vi "Valuta procedure start stop.vi"(6 "UTILIZZO BANCO":T1(ring), 7 "Modalità avvio":T9={"MODALITA' BANCO"=enum."ALIMENTATORE E FRENO", "MODALITA' AVVIO MOTORE"=enum."AVVIO A TENSIONE RIDOTTA", "MODALITA' AVVIO FRENO"=enum."MARCIA PRIMA AVVIO", "V avvio[V]"=0.0, "F avvio[Hz]"=0.0, "%V ridotta"=0.0, "C avvio [Nm]"=0.0, "RPM avvio"=0.0, "SERVO AVVIO"=FALSE, "SENSO DI ROTAZIONE"=FALSE}, 8 "Stato alimentatore 1":T6 {"Alimentatore 1"."Status ref"."RIF 2" scale=0.0..100.0; "Alimentatore 1"."Status ref"."RIF 1" scale=0.0..100.0}, 9 "Stato inverter":T7, 10 "NUOVO STEP":T3={"Tipo prova"="", "Misura resistenza ?"=FALSE, "Tempo Step[s]"=1.0, "Freno"={"MARCIA"=FALSE, "Control Type"=enum."Speed [RPM]", "RIF %"=1.0}, "ALIMENTATORE 1"={"MARCIA"=FALSE, "RIF V"=1.0, "RIF F"=1.0}, "ALIMENTATORE 2"={"MARCIA"=FALSE, "RIF V"=0.0, "RIF F"=0.0}, "Caratteristiche step"={"Attendi stabilizz."=FALSE, "Acq. fine step?"=FALSE, "Acq. automatiche"=FALSE, "PID FRENO"=FALSE, "PID ALIMENTATORE 1"=FALSE, "PID ALIMENTATORE 2"=FALSE, "CAMBIA PROVA SE EQ. TERMICO"=FALSE}} {"Tempo Step[s]" format="%#.1f"}, 11 "Cluster":T2) -> (3 "Prosegui":bool=TRUE)   [LabVIEW 2019]
uses:
  TypeDef/Stato inverter selezionato.ctl
  TypeDef/Comandi freno.ctl
  TypeDef/Comandi_Alimentatore.ctl
  GESTIONE PROFILI Folder/controls/STEP.ctl
  GESTIONE PROFILI Folder/controls/Caratteristiche step.ctl
  TypeDef/PROCEDURE.ctl
  Global Fine procedure.vi
panel:
  # "CHANGING CONTROL\nTYPE...."
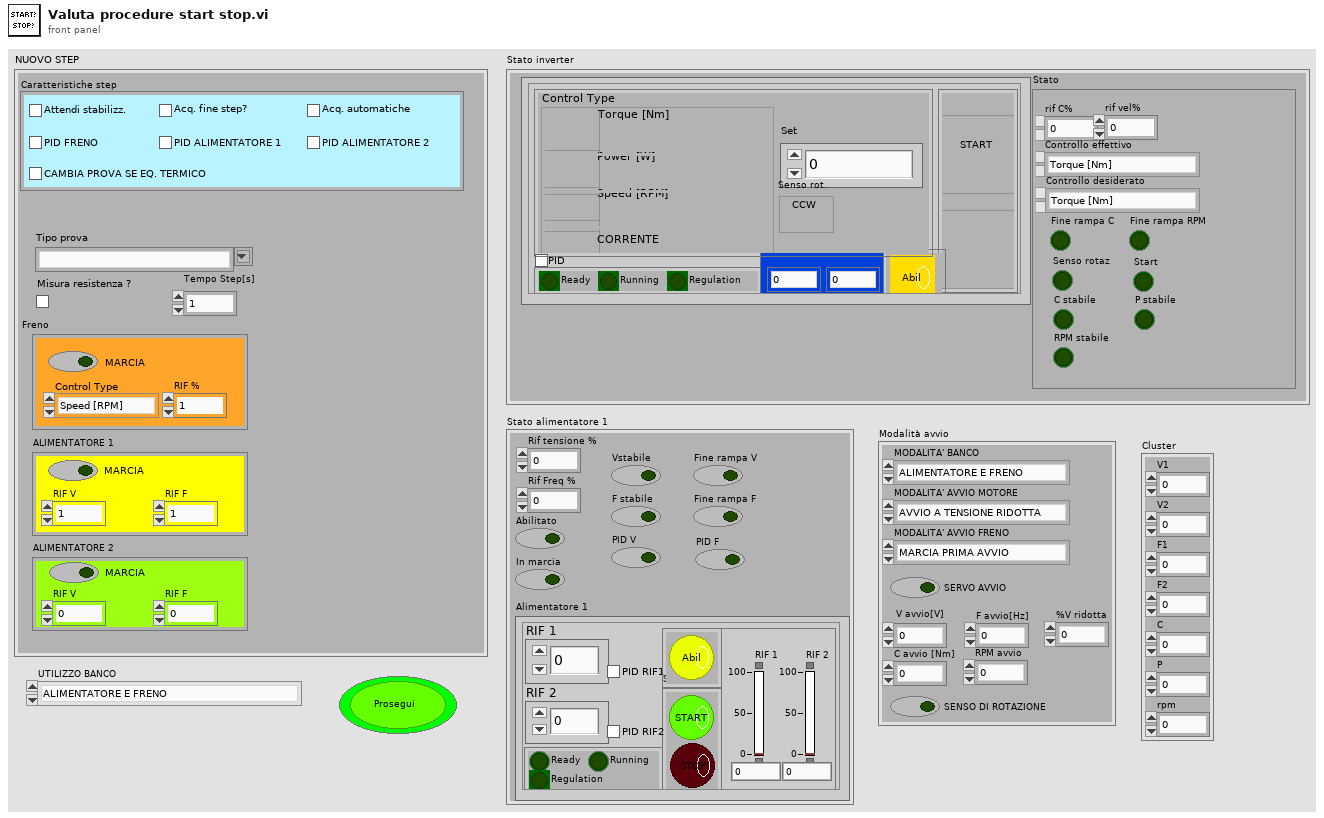
[diagram p1: front panel]
types:
  T1 = enum32{"ALIMENTATORE E FRENO", "SOLO ALIMENTATORE", "SOLO FRENO (TRASCINAMENTO)", "GESTIONE MANUALE", "SOLO ACQUISITORE", "VARIAC"}
  T2 = cluster{"V1":dbl, "V2":dbl, "F1":dbl, "F2":dbl, "C":dbl, "P":dbl, "rpm":dbl}
  T3 = typedef "STEP.ctl" = cluster{"Tipo prova":string, "Misura resistenza ?":bool, "Tempo Step[s]":dbl, "Freno":cluster{"MARCIA":bool, "Control Type":enum32{"Torque [Nm]", "Power [W]", "Speed [RPM]", "Corrente [A]"}, "RIF %":dbl}, "ALIMENTATORE 1":cluster{"MARCIA":bool, "RIF V":dbl, "RIF F":dbl}, "ALIMENTATORE 2":cluster{"MARCIA":bool, "RIF V":dbl, "RIF F":dbl}, "Caratteristiche step":T4}
  T4 = typedef "Caratteristiche step.ctl" = cluster{"Attendi stabilizz.":bool, "Acq. fine step?":bool, "Acq. automatiche":bool, "PID FRENO":bool, "PID ALIMENTATORE 1":bool, "PID ALIMENTATORE 2":bool, "CAMBIA PROVA SE EQ. TERMICO":bool}
  T5 = typedef "Comandi_Alimentatore.ctl" = cluster{"RIF 1":dbl, "RIF 2":dbl, "Status":cluster{"Ready":bool, "Running":bool, "Regulation":bool}, "Start\\stop":cluster{"Start":bool, "Stop":bool}, "PID RIF1":bool, "PID RIF2":bool, "Status ref":cluster{"RIF 1":dbl, "RIF 2":dbl}, "Abilita":cluster{"Abilita":bool}}
  T6 = cluster{"Rif tensione %":dbl, "Rif Freq %":dbl, "Abilitato":bool, "In marcia":bool, "Fine rampa V":bool, "Fine rampa F":bool, "Vstabile":bool, "F stabile":bool, "PID V":bool, "PID F":bool, "Alimentatore 1":T5}
  T7 = typedef "Stato inverter selezionato.ctl" = cluster{"Stato comandi freno":T8, "Stato":cluster{"rif C%":dbl, "rif vel%":dbl, "Controllo effettivo":enum32{"Torque [Nm]", "Power [W]", "Speed [RPM]"}, "Controllo desiderato":enum32{"Torque [Nm]", "Power [W]", "Speed [RPM]"}, "Fine rampa C":bool, "Fine rampa RPM":bool, "Senso rotaz":bool, "Start":bool, "C stabile":bool, "P stabile":bool, "RPM stabile":bool}}
  T8 = typedef "Comandi freno.ctl" = cluster{"Control":cluster{"Control Type":enum32{"Torque [Nm]", "Power [W]", "Speed [RPM]", "Corrente [A]"}, "Set":dbl, "Inverti senso di rotazione":bool}, "Start\\stop":cluster{"Start":bool, "STOP":bool}, "Status":cluster{"Ready":bool, "Running":bool, "Regulation":bool}, "PID":bool, "Abilita":cluster{"Abilita":bool}, "Status ref":cluster{"Torque":dbl, "Speed":dbl}}
  T9 = typedef "Modalità avvio.ctl" = cluster{"MODALITA' BANCO":enum32{"ALIMENTATORE E FRENO", "SOLO ALIMENTATORE", "SOLO FRENO", "GESTIONE MANUALE", "SOLO ACQUISITORE", "VARIAC"}, "MODALITA' AVVIO MOTORE":enum32{"AVVIO A TENSIONE RIDOTTA", "AVVIO IN RAMPA", "AVVIO DIRETTO DA ALIM", "AVVIO DIRETTO DA LINEA"}, "MODALITA' AVVIO FRENO":enum32{"MARCIA DOPO AVVIO MOTORE", "MARCIA PRIMA AVVIO"}, "V avvio[V]":dbl, "F avvio[Hz]":dbl, "%V ridotta":dbl, "C avvio [Nm]":dbl, "RPM avvio":dbl, "SERVO AVVIO":bool, "SENSO DI ROTAZIONE":bool}
  T10 = typedef "PROCEDURE.ctl" = enum16{"START", "STOP AUTOMATICO", "STOP FRENO", "ABILITA POTENZA", "DISABILITA POTENZA", "CHIUDI POTENZA", "APRI POTENZA", "MISURA RESISTENZA RESISTOMAT", "PROVA ROTORE BLOCCATO", "MISURA RESISTENZA RES METER", "START AFE ALTERNATORI", "STOP AFE ALTERNATORI", "STOP ALIMENTATORE", "CONFIG CONTROLLO FRENO", "ALLARME", "START PROFILO", "SVUOTA BUFFER PROCEDURE E OPERAZIONI"}
  T11 = cluster{"Message":string, "Message Data":variant}
  T12 = enum32{"ALIMENTATORE E FRENO", "SOLO ALIMENTATORE", "SOLO FRENO", "GESTIONE MANUALE"}
  T13 = enum32{"ALIMENTATORE E FRENO", "SOLO ALIMENTATORE", "SOLO FRENO", "GESTIONE MANUALE", "SOLO ACQUISITORE", "VARIAC"}
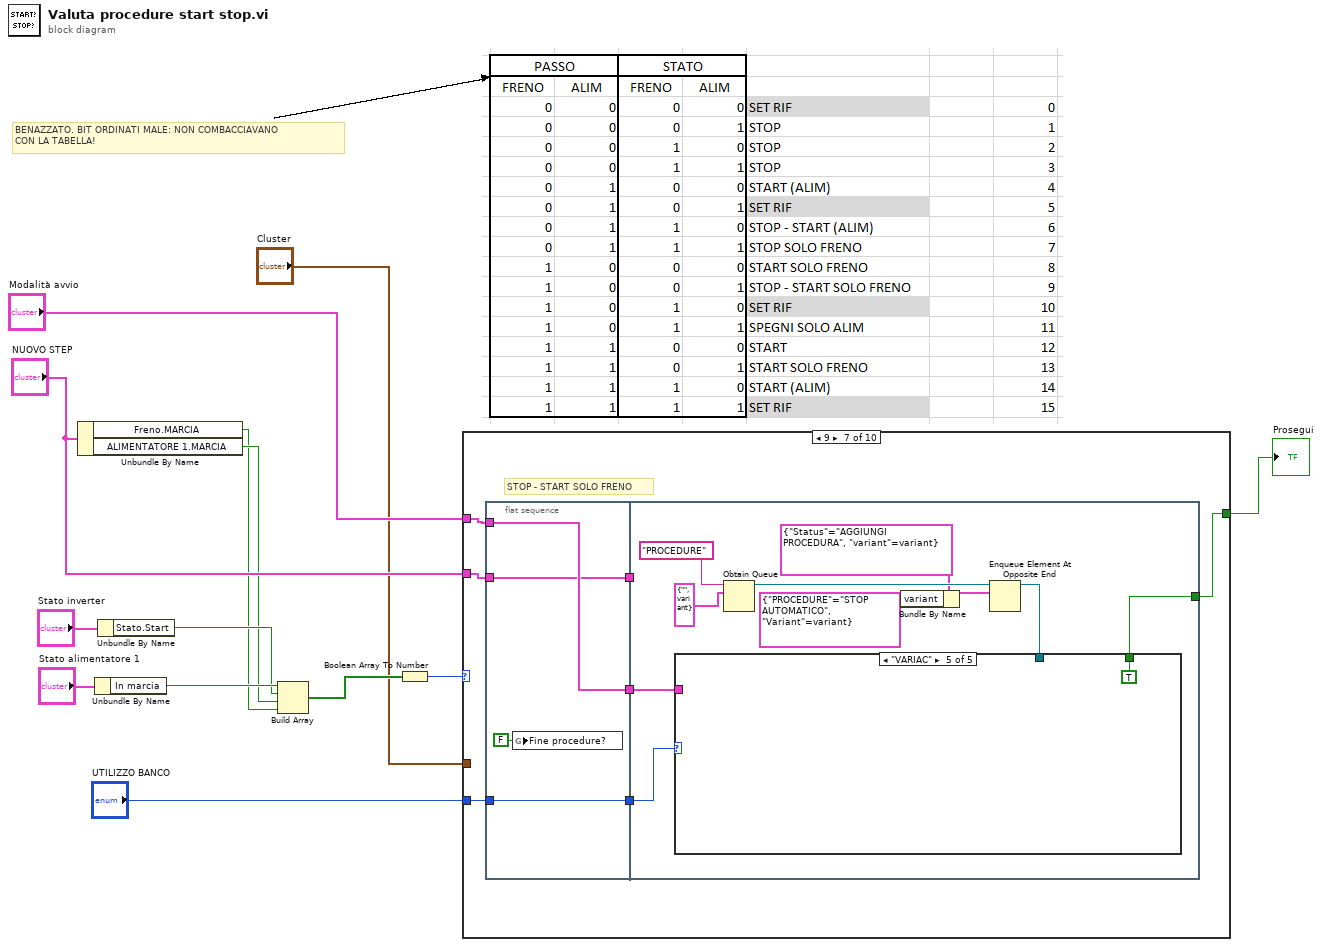
[diagram p0: block diagram]
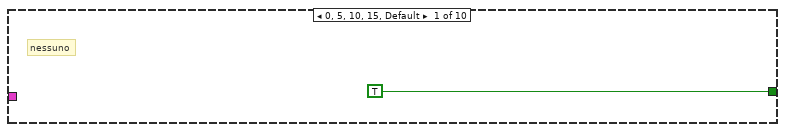
[diagram p2: hidden frame]
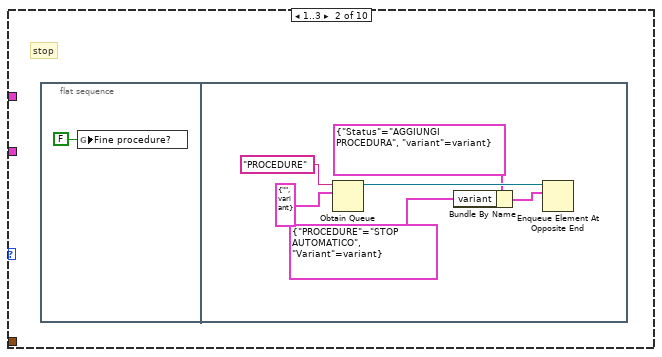
[diagram p3: hidden frame]
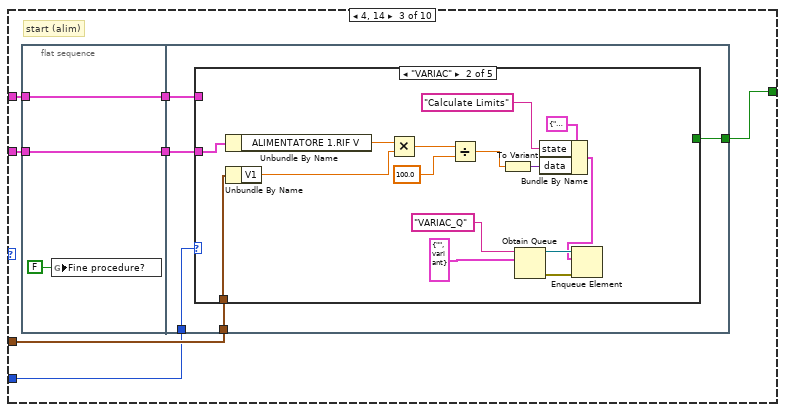
[diagram p4: hidden frame]
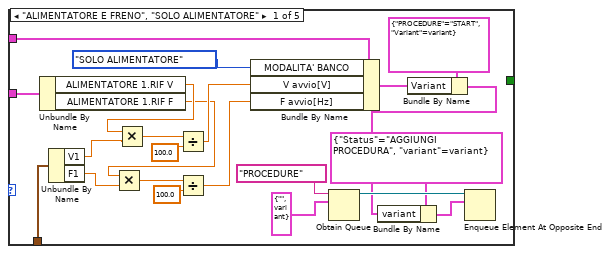
[diagram p5: hidden frame]
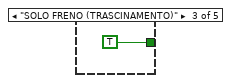
[diagram p6: hidden frame]
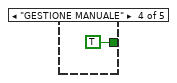
[diagram p7: hidden frame]
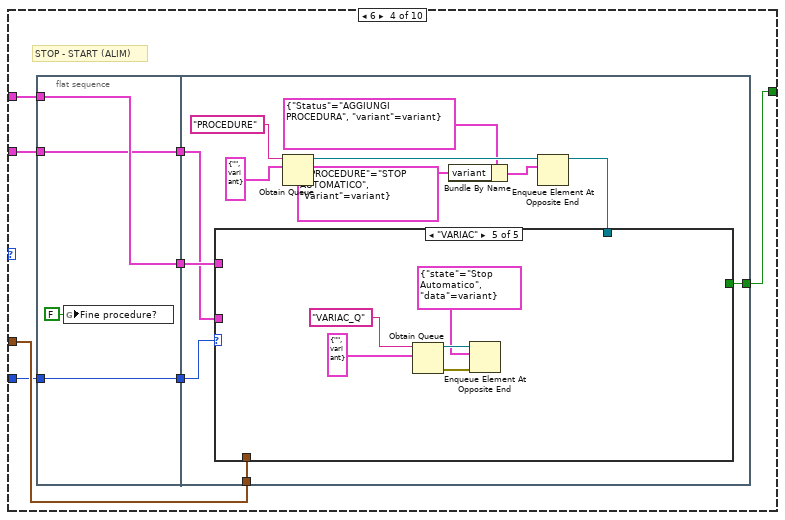
[diagram p9: hidden frame]
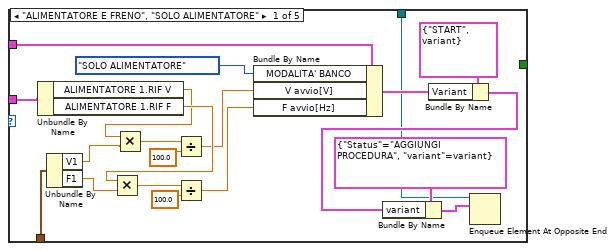
[diagram p10: hidden frame]
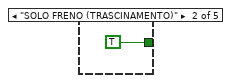
[diagram p11: hidden frame]
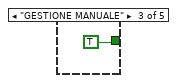
[diagram p12: hidden frame]
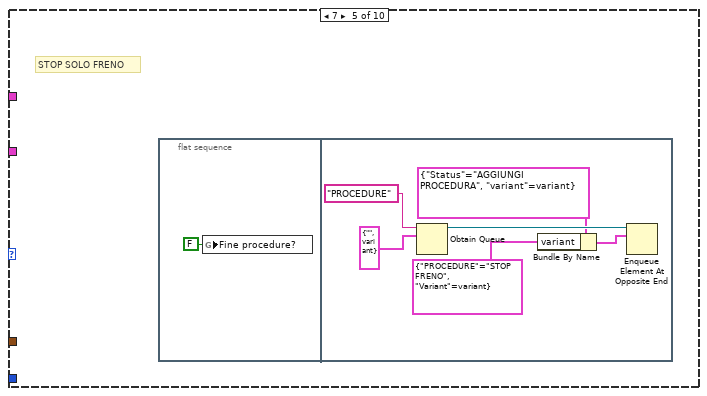
[diagram p14: hidden frame]
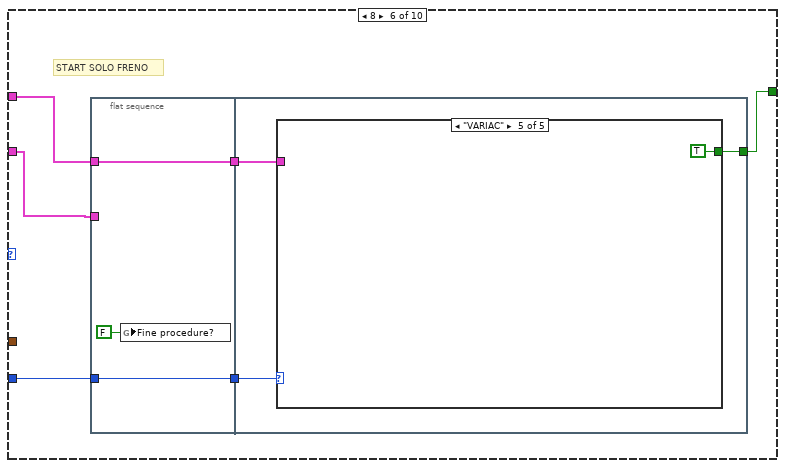
[diagram p15: hidden frame]
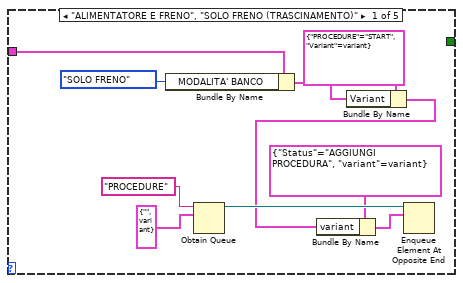
[diagram p16: hidden frame]
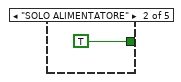
[diagram p17: hidden frame]
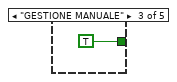
[diagram p18: hidden frame]
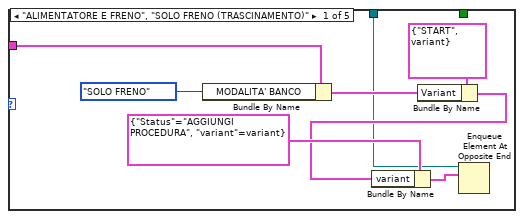
[diagram p20: hidden frame]
diagram:
  # "BENAZZATO. BIT ORDINATI MALE: NON COMBACCIAVANO\nCON LA TABELLA!"
  n1 = Unbundle By Name("NUOVO STEP") -> ("Freno.MARCIA"=w1:bool, "ALIMENTATORE 1.MARCIA"=w2:bool)
  n2 = Unbundle By Name("Stato alimentatore 1") -> ("In marcia"=w4:bool)
  n3 = Unbundle By Name("Stato inverter") -> ("Stato.Start"=w3:bool)
  n4 = Build Array(w4, w3, w2, w1) -> (w13:bool[])
  n5 = Boolean Array To Number(Boolean array=w13) -> (number=w5:u32)
  n6 = case shown="9" w5 {
    tunnel: [TRUE ("Prosegui") _ w22 w76 _ w134 w159 TRUE ("Prosegui") w192 w276] -> w12
    tunnel: "Modalità avvio" -> [_ _ w28 w82 _ w138 w163 _ w197 w280]
    tunnel: "NUOVO STEP" -> [_ _ w27 w80 _ w137 w162 _ w196 w279]
    tunnel: "Cluster" -> [_ _ w24 w79 _ _ _ _ w195 _]
    tunnel: "UTILIZZO BANCO" -> [_ _ w23 w77 _ w135 w160 _ w193 w277]
    frame 0, 5, 10, 15, Default {
      # "nessuno"
    }
    frame 1..3 {
      # "stop"
      n7 = flat-sequence {
        frame #0 {
          n8 = global write "Global Fine procedure.vi" "Fine procedure?"(FALSE ("Fine procedure?")) -> ()
        }
        frame #1 {
          n9 = Obtain Queue(name (unnamed)="PROCEDURE", element data type=T11 {"Message"="", "Message Data"=variant} ("Message Cluster")) -> (queue out=w21:refnum<queue>)  [unwired: 3 in, 2 out]
          n10 = Bundle By Name(cluster=cluster{"Status":string, "variant":variant} {"Status"="AGGIUNGI PROCEDURA", "variant"=variant}, "variant"=cluster{"PROCEDURE":T10, "Variant":variant} {"PROCEDURE"=enum."STOP AUTOMATICO", "Variant"=variant}) -> (w19:cluster{"Status":string, "variant":variant})
          n11 = Enqueue Element At Opposite End(queue=w21, element=w19) -> ()  [unwired: 2 in, 3 out]
        }
      }
    }
    frame 4, 14 {
      # "start (alim)"
      n12 = flat-sequence {
        tunnel: w27 -> [w30]
        tunnel: w28 -> [w31]
        tunnel: [w31] -> w26
        tunnel: [w30] -> w25
        tunnel: w26 -> [w36]
        tunnel: w25 -> [w35]
        tunnel: w24 -> [w34]
        tunnel: w23 -> [w33]
        tunnel: [w32] -> w22
        frame #0 {
          n13 = global write "Global Fine procedure.vi" "Fine procedure?"(FALSE ("Fine procedure?")) -> ()
        }
        frame #1 {
          n14 = case shown="\"VARIAC\"" w33 {
            tunnel: w36 -> [w58 _ _ _ _]
            tunnel: w35 -> [w56 w73 _ _ _]
            tunnel: w34 -> [w48 w72 _ _ _]
            tunnel: [_ _ TRUE TRUE _] -> w32
            frame "ALIMENTATORE E FRENO", "SOLO ALIMENTATORE" {
              n15 = Unbundle By Name(w56) -> ("ALIMENTATORE 1.RIF V"=w43:dbl, "ALIMENTATORE 1.RIF F"=w38:dbl)
              n16 = Unbundle By Name(w48) -> ("V1"=w44:dbl, "F1"=w40:dbl)
              n17 = Multiply(x=w38, y=w40) -> (x*y=w39:dbl)
              n18 = Multiply(x=w43, y=w44) -> (x*y=w42:dbl)
              n19 = Divide(x=w42, y=100.0) -> (x/y=w41:dbl)
              n20 = Divide(x=w39, y=100.0) -> (x/y=w37:dbl)
              n21 = Bundle By Name(cluster=w58, "MODALITA' BANCO"=T12."SOLO ALIMENTATORE", "V avvio[V]"=w41, "F avvio[Hz]"=w37) -> (w49:T9)
              n22 = Obtain Queue(name (unnamed)="PROCEDURE", element data type=T11 {"Message"="", "Message Data"=variant} ("Message Cluster")) -> (queue out=w55:refnum<queue>)  [unwired: 3 in, 2 out]
              n23 = Bundle By Name(cluster=cluster{"PROCEDURE":T10, "Variant":variant} {"PROCEDURE"=enum."START", "Variant"=variant}, "Variant"=w49) -> (w47:cluster{"PROCEDURE":T10, "Variant":variant})
              n24 = Bundle By Name(cluster=cluster{"Status":string, "variant":variant} {"Status"="AGGIUNGI PROCEDURA", "variant"=variant}, "variant"=w47) -> (w53:cluster{"Status":string, "variant":variant})
              n25 = Enqueue Element At Opposite End(queue=w55, element=w53) -> ()  [unwired: 2 in, 3 out]
            }
            frame "VARIAC" {
              n26 = Unbundle By Name(w73) -> ("ALIMENTATORE 1.RIF V"=w69:dbl)
              n27 = Unbundle By Name(w72) -> ("V1"=w70:dbl)
              n28 = Multiply(x=w69, y=w70) -> (x*y=w68:dbl)
              n29 = Divide(x=w68, y=100.0) -> (x/y=w60:dbl)
              n30 = To Variant(anything=w60) -> (Variant=w61:variant)
              n31 = Obtain Queue(name (unnamed)="VARIAC_Q", element data type=cluster{"state":string, "data":variant} {"state"="", "data"=variant} ("element")) -> (queue out=w65:refnum<queue>, error out=w64:errorcluster)  [unwired: 3 in, 1 out]
              n32 = Bundle By Name(cluster=cluster{"state":string, "data":variant} {"state"="", "data"=variant} ("element"), "state"="Calculate Limits", "data"=w61) -> (w59:cluster{"state":string, "data":variant})
              n33 = Enqueue Element(queue=w65, element=w59, error in (no error)=w64) -> ()  [unwired: 1 in, 3 out]
            }
            frame "SOLO FRENO (TRASCINAMENTO)" {
            }
            frame "GESTIONE MANUALE" {
            }
            frame "SOLO ACQUISITORE" {
            }
          }
        }
      }
    }
    frame 6 {
      # "STOP - START (ALIM)"
      n34 = flat-sequence {
        tunnel: [w86] -> w83
        tunnel: w82 -> [w86]
        tunnel: [w85] -> w81
        tunnel: w80 -> [w85]
        tunnel: [w84] -> w78
        tunnel: w77 -> [w84]
        tunnel: w83 -> [w93]
        tunnel: w81 -> [w91]
        tunnel: w79 -> [w90]
        tunnel: w78 -> [w89]
        tunnel: [w88] -> w76
        frame #0 {
          n35 = global write "Global Fine procedure.vi" "Fine procedure?"(FALSE ("Fine procedure?")) -> ()
        }
        frame #1 {
          n36 = Obtain Queue(name (unnamed)="PROCEDURE", element data type=T11 {"Message"="", "Message Data"=variant} ("Message Cluster")) -> (queue out=w99:refnum<queue>)  [unwired: 3 in, 2 out]
          n37 = Bundle By Name(cluster=cluster{"Status":string, "variant":variant} {"Status"="AGGIUNGI PROCEDURA", "variant"=variant}, "variant"=cluster{"PROCEDURE":T10, "Variant":variant} {"PROCEDURE"=enum."STOP AUTOMATICO", "Variant"=variant}) -> (w97:cluster{"Status":string, "variant":variant})
          n38 = Enqueue Element At Opposite End(queue=w99, element=w97) -> (queue out=w92:refnum<queue>)  [unwired: 2 in, 2 out]
          n39 = case shown="\"VARIAC\"" w89 {
            tunnel: w93 -> [w113 _ _ _ _]
            tunnel: w92 -> [w112 _ _ _ _]
            tunnel: w91 -> [w105 _ _ _ _]
            tunnel: w90 -> [w100 _ _ _ _]
            tunnel: [_ TRUE TRUE _ _] -> w88
            frame "ALIMENTATORE E FRENO", "SOLO ALIMENTATORE" {
              n40 = Unbundle By Name(w105) -> ("ALIMENTATORE 1.RIF V"=w103:dbl, "ALIMENTATORE 1.RIF F"=w104:dbl)
              n41 = Unbundle By Name(w100) -> ("V1"=w109:dbl, "F1"=w107:dbl)
              n42 = Multiply(x=w104, y=w107) -> (x*y=w106:dbl)
              n43 = Multiply(x=w103, y=w109) -> (x*y=w108:dbl)
              n44 = Divide(x=w108, y=100.0) -> (x/y=w101:dbl)
              n45 = Divide(x=w106, y=100.0) -> (x/y=w102:dbl)
              n46 = Bundle By Name(cluster=w113, "MODALITA' BANCO"=T12."SOLO ALIMENTATORE", "V avvio[V]"=w101, "F avvio[Hz]"=w102) -> (w115:T9)
              n47 = Bundle By Name(cluster=cluster{"PROCEDURE":T10, "Variant":variant} {"PROCEDURE"=enum."START", "Variant"=variant}, "Variant"=w115) -> (w114:cluster{"PROCEDURE":T10, "Variant":variant})
              n48 = Bundle By Name(cluster=cluster{"Status":string, "variant":variant} {"Status"="AGGIUNGI PROCEDURA", "variant"=variant}, "variant"=w114) -> (w117:cluster{"Status":string, "variant":variant})
              n49 = Enqueue Element At Opposite End(queue=w112, element=w117) -> ()  [unwired: 2 in, 3 out]
            }
            frame "SOLO FRENO (TRASCINAMENTO)" {
            }
            frame "GESTIONE MANUALE" {
            }
            frame "SOLO ACQUISITORE" {
            }
            frame "VARIAC" {
              n50 = Obtain Queue(name (unnamed)="VARIAC_Q", element data type=cluster{"state":string, "data":variant} {"state"="", "data"=variant} ("element")) -> (queue out=w126:refnum<queue>, error out=w125:errorcluster)  [unwired: 3 in, 1 out]
              n51 = Enqueue Element At Opposite End(queue=w126, element=cluster{"state":string, "data":variant} {"state"="Stop Automatico", "data"=variant}, error in (no error)=w125) -> ()  [unwired: 1 in, 3 out]
            }
          }
        }
      }
    }
    frame 7 {
      # "STOP SOLO FRENO"
      n52 = flat-sequence {
        frame #0 {
          n53 = global write "Global Fine procedure.vi" "Fine procedure?"(FALSE ("Fine procedure?")) -> ()
        }
        frame #1 {
          n54 = Obtain Queue(name (unnamed)="PROCEDURE", element data type=T11 {"Message"="", "Message Data"=variant} ("Message Cluster")) -> (queue out=w133:refnum<queue>)  [unwired: 3 in, 2 out]
          n55 = Bundle By Name(cluster=cluster{"Status":string, "variant":variant} {"Status"="AGGIUNGI PROCEDURA", "variant"=variant}, "variant"=cluster{"PROCEDURE":T10, "Variant":variant} {"PROCEDURE"=enum."STOP FRENO", "Variant"=variant}) -> (w131:cluster{"Status":string, "variant":variant})
          n56 = Enqueue Element At Opposite End(queue=w133, element=w131) -> ()  [unwired: 2 in, 3 out]
        }
      }
    }
    frame 8 {
      # "START SOLO FRENO"
      n57 = flat-sequence {
        tunnel: w137 -> [_]
        tunnel: w138 -> [w142]
        tunnel: [w142] -> w139
        tunnel: [w140] -> w136
        tunnel: w135 -> [w140]
        tunnel: w139 -> [w145]
        tunnel: w136 -> [w144]
        tunnel: [w143] -> w134
        frame #0 {
          n58 = global write "Global Fine procedure.vi" "Fine procedure?"(FALSE ("Fine procedure?")) -> ()
        }
        frame #1 {
          n59 = case shown="\"VARIAC\"" w144 {
            tunnel: w145 -> [w155 _ _ _ _]
            tunnel: [_ TRUE TRUE _ TRUE] -> w143
            frame "ALIMENTATORE E FRENO", "SOLO FRENO (TRASCINAMENTO)" {
              n60 = Bundle By Name(cluster=w155, "MODALITA' BANCO"=T12."SOLO FRENO") -> (w147:T9)
              n61 = Obtain Queue(name (unnamed)="PROCEDURE", element data type=T11 {"Message"="", "Message Data"=variant} ("Message Cluster")) -> (queue out=w153:refnum<queue>)  [unwired: 3 in, 2 out]
              n62 = Bundle By Name(cluster=cluster{"PROCEDURE":T10, "Variant":variant} {"PROCEDURE"=enum."START", "Variant"=variant}, "Variant"=w147) -> (w146:cluster{"PROCEDURE":T10, "Variant":variant})
              n63 = Bundle By Name(cluster=cluster{"Status":string, "variant":variant} {"Status"="AGGIUNGI PROCEDURA", "variant"=variant}, "variant"=w146) -> (w151:cluster{"Status":string, "variant":variant})
              n64 = Enqueue Element At Opposite End(queue=w153, element=w151) -> ()  [unwired: 2 in, 3 out]
            }
            frame "SOLO ALIMENTATORE" {
            }
            frame "GESTIONE MANUALE" {
            }
            frame "SOLO ACQUISITORE" {
            }
            frame "VARIAC" {
            }
          }
        }
      }
    }
    frame 9 {
      # "STOP - START SOLO FRENO"
      n65 = flat-sequence {
        tunnel: [w168] -> w165
        tunnel: w163 -> [w168]
        tunnel: [w167] -> w164
        tunnel: w162 -> [w167]
        tunnel: [w166] -> w161
        tunnel: w160 -> [w166]
        tunnel: w165 -> [w173]
        tunnel: w164 -> [_]
        tunnel: w161 -> [w171]
        tunnel: [w170] -> w159
        frame #0 {
          n66 = global write "Global Fine procedure.vi" "Fine procedure?"(FALSE ("Fine procedure?")) -> ()
        }
        frame #1 {
          n67 = Obtain Queue(name (unnamed)="PROCEDURE", element data type=T11 {"Message"="", "Message Data"=variant} ("Message Cluster")) -> (queue out=w179:refnum<queue>)  [unwired: 3 in, 2 out]
          n68 = Bundle By Name(cluster=cluster{"Status":string, "variant":variant} {"Status"="AGGIUNGI PROCEDURA", "variant"=variant}, "variant"=cluster{"PROCEDURE":T10, "Variant":variant} {"PROCEDURE"=enum."STOP AUTOMATICO", "Variant"=variant}) -> (w177:cluster{"Status":string, "variant":variant})
          n69 = Enqueue Element At Opposite End(queue=w179, element=w177) -> (queue out=w172:refnum<queue>)  [unwired: 2 in, 2 out]
          n70 = case shown="\"VARIAC\"" w171 {
            tunnel: w173 -> [w181 _ _ _ _]
            tunnel: w172 -> [w180 _ _ _ _]
            tunnel: [_ TRUE TRUE _ TRUE] -> w170
            frame "ALIMENTATORE E FRENO", "SOLO FRENO (TRASCINAMENTO)" {
              n71 = Bundle By Name(cluster=w181, "MODALITA' BANCO"=T12."SOLO FRENO") -> (w183:T9)
              n72 = Bundle By Name(cluster=cluster{"PROCEDURE":T10, "Variant":variant} {"PROCEDURE"=enum."START", "Variant"=variant}, "Variant"=w183) -> (w182:cluster{"PROCEDURE":T10, "Variant":variant})
              n73 = Bundle By Name(cluster=cluster{"Status":string, "variant":variant} {"Status"="AGGIUNGI PROCEDURA", "variant"=variant}, "variant"=w182) -> (w185:cluster{"Status":string, "variant":variant})
              n74 = Enqueue Element At Opposite End(queue=w180, element=w185) -> ()  [unwired: 2 in, 3 out]
            }
            frame "SOLO ALIMENTATORE" {
            }
            frame "GESTIONE MANUALE" {
            }
            frame "SOLO ACQUISITORE" {
            }
            frame "VARIAC" {
            }
          }
        }
      }
    }
    frame 11 {
      # "SPEGNI SOLO ALIM"
    }
    frame 12 {
      # "START"
      n75 = flat-sequence {
        tunnel: w196 -> [w202]
        tunnel: w197 -> [w203]
        tunnel: [w203] -> w199
        tunnel: [w202] -> w198
        tunnel: [w200] -> w194
        tunnel: w193 -> [w200]
        tunnel: w199 -> [w208]
        tunnel: w198 -> [w207]
        tunnel: w195 -> [w206]
        tunnel: w194 -> [w205]
        tunnel: [w204] -> w192
        frame #0 {
          n76 = global write "Global Fine procedure.vi" "Fine procedure?"(FALSE ("Fine procedure?")) -> ()
        }
        frame #1 {
          n77 = case shown="\"SOLO FRENO (TRASCINAMENTO)\"" w205 {
            tunnel: w208 -> [w230 w252 w274 _]
            tunnel: w207 -> [w213 w235 w256 _]
            tunnel: w206 -> [w210 w232 w253 _]
            tunnel: [_ _ _ TRUE] -> w204
            frame "ALIMENTATORE E FRENO", Default {
              n78 = Unbundle By Name(w213) -> ("ALIMENTATORE 1.RIF V"=w218:dbl, "ALIMENTATORE 1.RIF F"=w214:dbl)
              n79 = Unbundle By Name(w210) -> ("V1"=w219:dbl, "F1"=w216:dbl)
              n80 = Multiply(x=w214, y=w216) -> (x*y=w215:dbl)
              n81 = Multiply(x=w218, y=w219) -> (x*y=w217:dbl)
              n82 = Divide(x=w217, y=100.0) -> (x/y=w212:dbl)
              n83 = Divide(x=w215, y=100.0) -> (x/y=w211:dbl)
              n84 = Bundle By Name(cluster=w230, "MODALITA' BANCO"=T13."ALIMENTATORE E FRENO", "V avvio[V]"=w212, "F avvio[Hz]"=w211) -> (w223:T9)
              n85 = Obtain Queue(name (unnamed)="PROCEDURE", element data type=T11 {"Message"="", "Message Data"=variant} ("Message Cluster")) -> (queue out=w229:refnum<queue>)  [unwired: 3 in, 2 out]
              n86 = Bundle By Name(cluster=cluster{"PROCEDURE":T10, "Variant":variant} {"PROCEDURE"=enum."START", "Variant"=variant}, "Variant"=w223) -> (w222:cluster{"PROCEDURE":T10, "Variant":variant})
              n87 = Bundle By Name(cluster=cluster{"Status":string, "variant":variant} {"Status"="AGGIUNGI PROCEDURA", "variant"=variant}, "variant"=w222) -> (w227:cluster{"Status":string, "variant":variant})
              n88 = Enqueue Element At Opposite End(queue=w229, element=w227) -> ()  [unwired: 2 in, 3 out]
            }
            frame "SOLO ALIMENTATORE" {
              n89 = Unbundle By Name(w235) -> ("ALIMENTATORE 1.RIF V"=w240:dbl, "ALIMENTATORE 1.RIF F"=w236:dbl)
              n90 = Unbundle By Name(w232) -> ("V1"=w241:dbl, "F1"=w238:dbl)
              n91 = Multiply(x=w236, y=w238) -> (x*y=w237:dbl)
              n92 = Multiply(x=w240, y=w241) -> (x*y=w239:dbl)
              n93 = Divide(x=w239, y=100.0) -> (x/y=w234:dbl)
              n94 = Divide(x=w237, y=100.0) -> (x/y=w233:dbl)
              n95 = Bundle By Name(cluster=w252, "MODALITA' BANCO"=T13."SOLO ALIMENTATORE", "V avvio[V]"=w234, "F avvio[Hz]"=w233) -> (w245:T9)
              n96 = Obtain Queue(name (unnamed)="PROCEDURE", element data type=T11 {"Message"="", "Message Data"=variant} ("Message Cluster")) -> (queue out=w251:refnum<queue>)  [unwired: 3 in, 2 out]
              n97 = Bundle By Name(cluster=cluster{"PROCEDURE":T10, "Variant":variant} {"PROCEDURE"=enum."START", "Variant"=variant}, "Variant"=w245) -> (w244:cluster{"PROCEDURE":T10, "Variant":variant})
              n98 = Bundle By Name(cluster=cluster{"Status":string, "variant":variant} {"Status"="AGGIUNGI PROCEDURA", "variant"=variant}, "variant"=w244) -> (w249:cluster{"Status":string, "variant":variant})
              n99 = Enqueue Element At Opposite End(queue=w251, element=w249) -> ()  [unwired: 2 in, 3 out]
            }
            frame "SOLO FRENO (TRASCINAMENTO)" {
              n100 = Unbundle By Name(w256) -> ("ALIMENTATORE 1.RIF V"=w261:dbl, "ALIMENTATORE 1.RIF F"=w257:dbl)
              n101 = Unbundle By Name(w253) -> ("V1"=w262:dbl, "F1"=w259:dbl)
              n102 = Multiply(x=w257, y=w259) -> (x*y=w258:dbl)
              n103 = Multiply(x=w261, y=w262) -> (x*y=w260:dbl)
              n104 = Divide(x=w260, y=100.0) -> (x/y=w255:dbl)
              n105 = Divide(x=w258, y=100.0) -> (x/y=w254:dbl)
              n106 = Bundle By Name(cluster=w274, "MODALITA' BANCO"=T12."SOLO FRENO", "V avvio[V]"=w255, "F avvio[Hz]"=w254) -> (w266:T9)
              n107 = Obtain Queue(name (unnamed)="PROCEDURE", element data type=T11 {"Message"="", "Message Data"=variant} ("Message Cluster")) -> (queue out=w272:refnum<queue>)  [unwired: 3 in, 2 out]
              n108 = Bundle By Name(cluster=cluster{"PROCEDURE":T10, "Variant":variant} {"PROCEDURE"=enum."START", "Variant"=variant}, "Variant"=w266) -> (w265:cluster{"PROCEDURE":T10, "Variant":variant})
              n109 = Bundle By Name(cluster=cluster{"Status":string, "variant":variant} {"Status"="AGGIUNGI PROCEDURA", "variant"=variant}, "variant"=w265) -> (w270:cluster{"Status":string, "variant":variant})
              n110 = Enqueue Element At Opposite End(queue=w272, element=w270) -> ()  [unwired: 2 in, 3 out]
            }
            frame "GESTIONE MANUALE" {
            }
          }
        }
      }
    }
    frame 13 {
      # "START SOLO FRENO"
      n111 = flat-sequence {
        tunnel: w279 -> [w285]
        tunnel: w280 -> [w286]
        tunnel: [w286] -> w282
        tunnel: [w285] -> w281
        tunnel: [w283] -> w278
        tunnel: w277 -> [w283]
        tunnel: w282 -> [w289]
        tunnel: w281 -> [_]
        tunnel: w278 -> [w288]
        tunnel: [w287] -> w276
        frame #0 {
          n112 = global write "Global Fine procedure.vi" "Fine procedure?"(FALSE ("Fine procedure?")) -> ()
        }
        frame #1 {
          n113 = case shown="\"VARIAC\"" w288 {
            tunnel: w289 -> [w299 _ _ _ _]
            tunnel: [_ TRUE TRUE _ _] -> w287
            frame "ALIMENTATORE E FRENO", "SOLO FRENO (TRASCINAMENTO)" {
              n114 = Bundle By Name(cluster=w299, "MODALITA' BANCO"=T12."SOLO FRENO") -> (w291:T9)
              n115 = Obtain Queue(name (unnamed)="PROCEDURE", element data type=T11 {"Message"="", "Message Data"=variant} ("Message Cluster")) -> (queue out=w297:refnum<queue>)  [unwired: 3 in, 2 out]
              n116 = Bundle By Name(cluster=cluster{"PROCEDURE":T10, "Variant":variant} {"PROCEDURE"=enum."START", "Variant"=variant}, "Variant"=w291) -> (w290:cluster{"PROCEDURE":T10, "Variant":variant})
              n117 = Bundle By Name(cluster=cluster{"Status":string, "variant":variant} {"Status"="AGGIUNGI PROCEDURA", "variant"=variant}, "variant"=w290) -> (w295:cluster{"Status":string, "variant":variant})
              n118 = Enqueue Element At Opposite End(queue=w297, element=w295) -> ()  [unwired: 2 in, 3 out]
            }
            frame "SOLO ALIMENTATORE" {
            }
            frame "GESTIONE MANUALE" {
            }
            frame "SOLO ACQUISITORE" {
            }
            frame "VARIAC" {
              # "DO NOTHING"
            }
          }
        }
      }
    }
  }
  "Prosegui" <- w12
